vi "Begin.vi"(8 "error in":errorcluster) -> (0 "error out":errorcluster)   [LabVIEW 2017]
doc: "Called before other user functions, this VI is expected to open initial I/O refnums, load in file data, and do all program initialization. Notice that the <B>error out</B> terminal is simply used for data flow. Wiring it to other structures or subVIs ensures that this VI runs first."
uses:
  <vilib>/Rock Robotics/WPI/DriverStation/WPI_DriverStationRobotMode2.ctl
  <vilib>/Rock Robotics/WPI/Joystick/WPI_JoystickDeviceEnum.ctl
  <vilib>/Rock Robotics/WPI/ThirdParty/Phoenix-LabVIEW/Motor Controller/Controls/CTRE_Phoenix_MotorControl_NeutralMode.ctl
  <vilib>/Rock Robotics/WPI/ThirdParty/Phoenix-LabVIEW/Motor Controller/Controls/CTRE_Phoenix_MotorControl_ControlMode.ctl
  <vilib>/Rock Robotics/SystemInterfaces/spilib/spi_bus.ctl
  <vilib>/Rock Robotics/WPI/ThirdParty/Phoenix-LabVIEW/Motor Controller/Controls/CTRE_Phoenix_MotorControl_FeedbackDevice.ctl
  <vilib>/Rock Robotics/WPI/Solenoid/WPI_SolenoidChannel.ctl
  <vilib>/Rock Robotics/WPI/Solenoid/WPI_SolenoidValue.ctl
  Robot Global Data.vi
  <vilib>/Rock Robotics/Network Tables/NT Write String Array.vi
  <vilib>/Rock Robotics/WPI/RobotDrive/WPI_RobotDriveOpen2MotorWithExistingMotors.vi
  <vilib>/Rock Robotics/WPI/Solenoid/WPI_SolenoidOpenDouble.vi
  <vilib>/Rock Robotics/WPI/Solenoid/WPI_SolenoidSetEnum.vi
  <vilib>/Rock Robotics/WPI/Utilities/WPI_GetSetVariantRefNum.vi
  <vilib>/Rock Robotics/Network Tables/NT Write String.vi
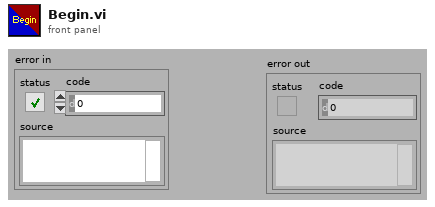
[diagram p1: front panel]
types:
  T1 = typedef "WPI_DriverStationRobotMode2.ctl" = enum16{"Autonomous Disabled", "Autonomous Enabled", "Teleop Disabled", "Teleop Enabled", "Disconnected", "Finish", "Test Disabled", "Test Enabled", "Emergency Stopped"}
  T2 = typedef "WPI_JoystickDeviceEnum.ctl" = enum16{"USB 0", "USB 1", "USB 2", "USB 3", "USB 4", "USB 5"}
  T3 = typedef "CTRE_Phoenix_MotorControl_NeutralMode.ctl" = enum8{"EEPROMSetting", "Override to Coast", "Override to Brake"}
  T4 = typedef "spi_bus.ctl" = enum16{"SPI On-Board, CS0", "SPI On-Board, CS1", "SPI On-Board, CS2", "SPI On-Board, CS3", "SPI MXP", "Invalid"}
  T5 = typedef "WPI_SolenoidValue.ctl" = enum16{"Off", "On", "Forward", "Reverse"}
  T6 = typedef "WPI_SolenoidChannel.ctl" = enum8{"Solenoid 0", "Solenoid 1", "Solenoid 2", "Solenoid 3", "Solenoid 4", "Solenoid 5", "Solenoid 6", "Solenoid 7", "Invalid"}
  T7 = typedef "WPI_JoystickDevRef.ctl" = cluster{"Device":T2}
  T8 = typedef "CTRE_Phoenix_MotorControl_ControlMode.ctl" = u16
  T9 = typedef "WPI_MotorControlDeviceRef.ctl" = cluster{"DeviceStatus":errorcluster, "Type":T10, "PWM":cluster{"PWM Channel":T11, "DeadBand":T12}, "CAN":cluster{"Device Number":u8, "SetOutput VI Ref":variant, "GetOutput VI Ref":variant, "Enable VI Ref":variant, "Disable VI Ref":variant, "Data":variant}, "Invert":bool, "DIO PWM":cluster{"PWM \"Enable\" Channel":T11, "DIOChannel":T13, "PWM Rate":dbl}}
  T10 = typedef "WPI_MotorControlType.ctl" = enum16{"PWM", "CAN", "DIO PWM"}
  T11 = typedef "FPGA_DIOPWMChannel.ctl" = enum8{"PWM 0", "PWM 1", "PWM 2", "PWM 3", "PWM 4", "PWM 5", "PWM 6", "PWM 7", "PWM 8", "PWM 9", "PWM MXP 0", "PWM MXP 1", "PWM MXP 2", "PWM MXP 3", "PWM MXP 4", "PWM MXP 5", "PWM MXP 6", "PWM MXP 7", "PWM MXP 8", "PWM MXP 9", "Invalid"}
  T12 = typedef "WPI_PWMDeadband.ctl" = cluster{"Name":string, "maxPositivePwm":i32, "minPositivePwm":i32, "centerPwm":i32, "maxNegativePwm":i32, "minNegativePwm":i32, "angularRange":u16}
  T13 = typedef "FPGA_DIOChannel.ctl" = enum8{"DIO 0", "DIO 1", "DIO 2", "DIO 3", "DIO 4", "DIO 5", "DIO 6", "DIO 7", "DIO 8", "DIO 9", "DIO MXP 0", "DIO MXP 1", "DIO MXP 2", "DIO MXP 3", "DIO MXP 4", "DIO MXP 5", "DIO MXP 6", "DIO MXP 7", "DIO MXP 8", "DIO MXP 9", "DIO MXP 10", "DIO MXP 11", "DIO MXP 12", "DIO MXP 13", "DIO MXP 14", "DIO MXP 15", "SPI Port CS1", "SPI Port CS2", "SPI Port CS3", "SPI Port MISO", "SPI Port MOSI", "Invalid"}
  T14 = typedef "WPI_RobotDriveDevRef.ctl" = cluster{"DevStatus":errorcluster, "Motors[]":T9[], "Square Inputs":bool, "Max Output":dbl}
  T15 = typedef "WPI_GyroDevRef.ctl" = cluster{"DevStatus":errorcluster, "Analog Channel":T16, "Gain (VoltsPerDegree/Second)":dbl, "Gyro Type":enum16{"Analog", "XRS450"}, "Handle":i32, "SPI Bus":T4, "Device Found":bool, "Sample Rate":dbl, "Calibrate On Open":bool, "Offset":dbl}
  T16 = typedef "FPGA_AIChannel.ctl" = enum8{"AI 0", "AI 1", "AI 2", "AI 3", "AI MXP 0", "AI MXP 1", "AI MXP 2", "AI MXP 3", "Invalid"}
  T17 = typedef "CTRE_Phoenix_MotorControl_FeedbackDevice.ctl" = i8
  T18 = typedef "WPI_SolenoidDevRef.ctl" = cluster{"DevStatus":errorcluster, "Pneumatics Control Module":u8, "Forward Solenoid Channel":T6, "Reverse Solenoid Channel":T6}
  T19 = typedef "WPI_CompressorDevRef.ctl" = cluster{"DevStatus":errorcluster, "Pneumatics Control Module":u8}
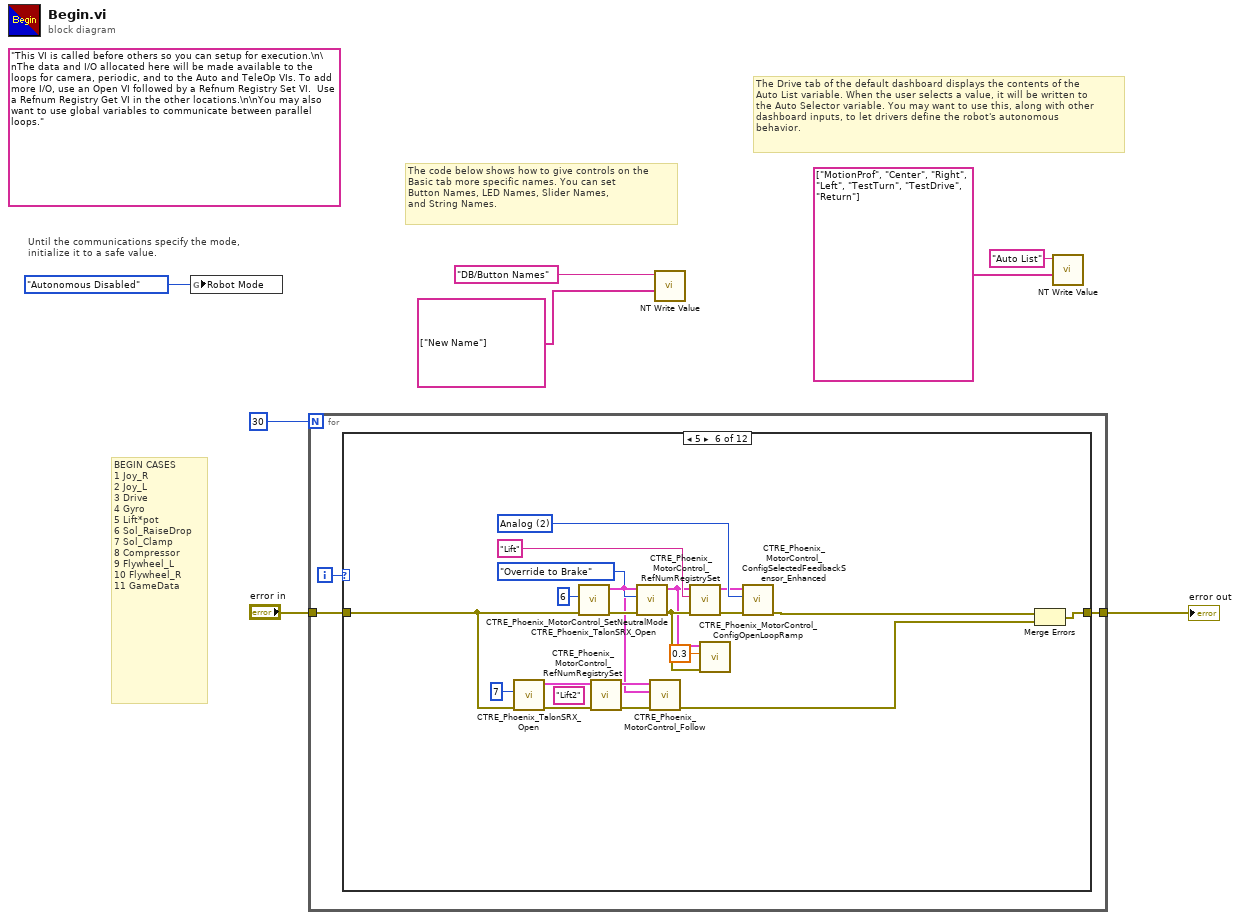
[diagram p0: block diagram]
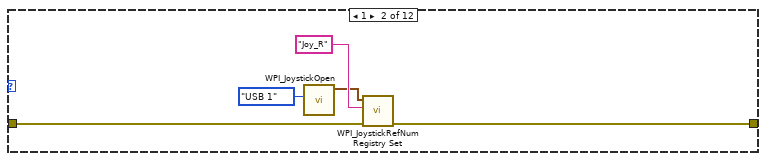
[diagram p3: hidden frame]
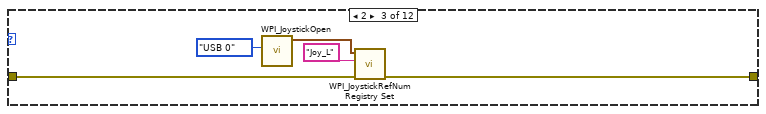
[diagram p4: hidden frame]
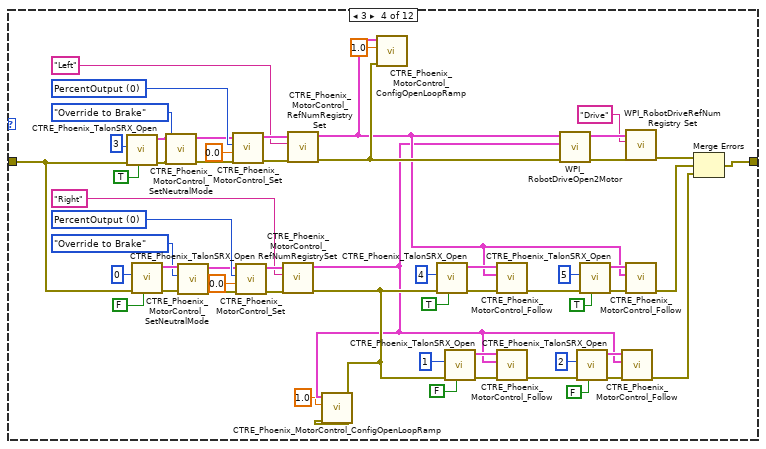
[diagram p5: hidden frame]
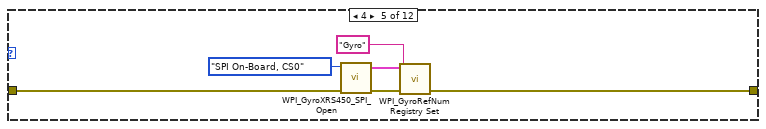
[diagram p6: hidden frame]
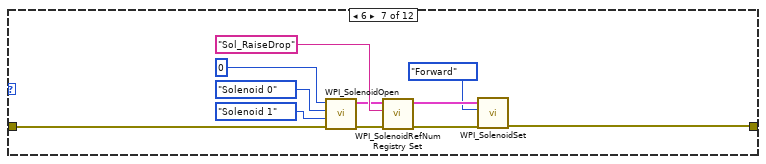
[diagram p7: hidden frame]
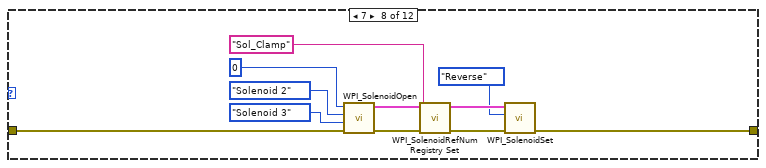
[diagram p8: hidden frame]
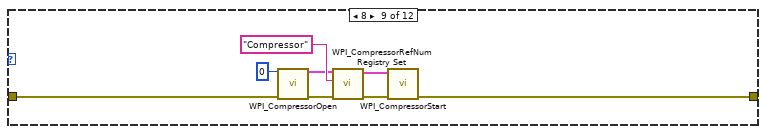
[diagram p9: hidden frame]
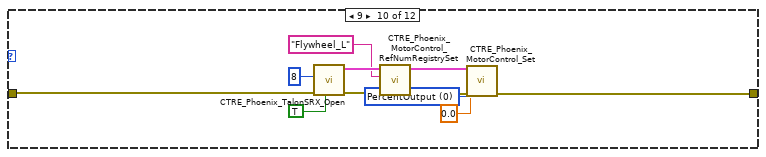
[diagram p10: hidden frame]
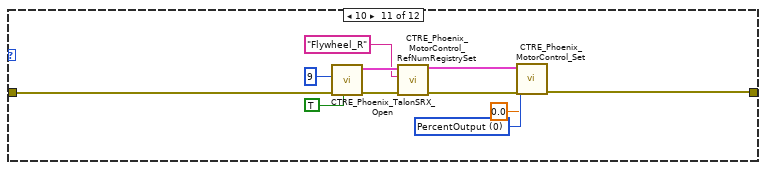
[diagram p11: hidden frame]
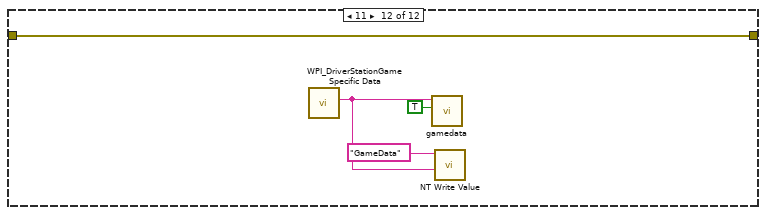
[diagram p12: hidden frame]
diagram:
  (unwired) "This VI is called before others so you can setup for execution.\n\nThe data and I/O allocated here will be made available to the loops for camera, periodic, and to the Auto and TeleOp VIs. To add more I/O, use an Open VI followed by a Refnum Registry Set VI.  Use a Refnum Registry Get VI in the other locations.\n\nYou may also want to use global variables to communicate between parallel loops."
  # "BEGIN CASES\n1 Joy_R\n2 Joy_L\n3 Drive\n4 Gyro\n5 Lift*pot\n6 Sol_RaiseDrop\n7 Sol_Clamp\n8 Compressor\n9 Flywheel_L\n10 Flywheel_R\n11 GameData"
  # "The Drive tab of the default dashboard displays the contents of the\nAuto List variable. When the user selects a value, it will be written to\nthe Auto Selector variable. You may want to use this, along with other\ndashboard inputs, to let drivers define the robot's autonomous\nbehavior."
  # "The code below shows how to give controls on the\nBasic tab more specific names. You can set\nButton Names, LED Names, Slider Names,\nand String Names."
  # "Until the communications specify the mode,\ninitialize it to a safe value."
  n1 = global write "Robot Global Data.vi" "Robot Mode"(WPI_DriverStationRobotMode2."Autonomous Disabled" ("Robot Mode")) -> ()
  n2 = for {
    N: 30 -> [_]
    tunnel: "error in" -> [w10]
    tunnel: [w9] -> w1
    i -> [w11]
    n3 = case shown="5" w11 {
      tunnel: w10 -> [w12 w16 w21 w39 w84 w86 w116 w122 w135 w146 w157 w161]
      tunnel: [w12 w15 w20 w78 w83 w87 w106 w118 w128 w139 w149 w161] -> w9
      frame 0, Default {
      }
      frame 1 {
        n4 = call <vilib>:"WPI_JoystickOpen.vi"("JoystickDevice"=WPI_JoystickDeviceEnum."USB 1") -> ("JoystickDevRef"=w14:T7)  [unwired: 10 in]
        n5 = call <vilib>:"WPI_JoystickRefNum Registry Set.vi"("error in (no error)"=w16, "refnum name"="Joy_R", "JoystickDevRef"=w14) -> ("error out"=w15:errorcluster)  [unwired: 7 in, 1 out]
      }
      frame 2 {
        n6 = call <vilib>:"WPI_JoystickOpen.vi"("JoystickDevice"=WPI_JoystickDeviceEnum."USB 0") -> ("JoystickDevRef"=w19:T7)  [unwired: 10 in]
        n7 = call <vilib>:"WPI_JoystickRefNum Registry Set.vi"("error in (no error)"=w21, "refnum name"="Joy_L", "JoystickDevRef"=w19) -> ("error out"=w20:errorcluster)  [unwired: 7 in, 1 out]
      }
      frame 3 {
        w61 = T8 0 items=["PercentOutput"=0, "Position"=1, "Velocity"=2, "Current"=3, "Follower"=5, "MotionProfile"=6, "MotionMagic"=7, "MotionMagicArc"=8, "MotionProfileArc"=10, "Disabled"=15] ("Control Mode")
        w71 = T8 0 items=["PercentOutput"=0, "Position"=1, "Velocity"=2, "Current"=3, "Follower"=5, "MotionProfile"=6, "MotionMagic"=7, "MotionMagicArc"=8, "MotionProfileArc"=10, "Disabled"=15] ("Control Mode")
        n8 = call <vilib>:"CTRE_Phoenix_TalonSRX_Open.vi"("Invert"=TRUE, "error in"=w39, "Device Number"=u8 3) -> ("error out"=w77:errorcluster, "CAN Talon SRX Ref"=w76:T9)  [unwired: 7 in]
        n9 = call <vilib>:"CTRE_Phoenix_TalonSRX_Open.vi"("Invert"=FALSE, "error in"=w39, "Device Number"=u8 0) -> ("error out"=w67:errorcluster, "CAN Talon SRX Ref"=w66:T9)  [unwired: 7 in]
        n10 = call <vilib>:"CTRE_Phoenix_MotorControl_SetNeutralMode.vi"("error in (no error)"=w77, "Motor Control Neutral Mode"=CTRE_Phoenix_MotorControl_NeutralMode."Override to Brake", "PhoenixMotorControlDevRef"=w76) -> ("error out"=w26:errorcluster, "PhoenixMotorControlDevRef"=w27:T9)  [unwired: 7 in]
        n11 = call <vilib>:"CTRE_Phoenix_MotorControl_SetNeutralMode.vi"("error in (no error)"=w67, "Motor Control Neutral Mode"=CTRE_Phoenix_MotorControl_NeutralMode."Override to Brake", "PhoenixMotorControlDevRef"=w66) -> ("error out"=w25:errorcluster, "PhoenixMotorControlDevRef"=w28:T9)  [unwired: 7 in]
        n12 = call <vilib>:"CTRE_Phoenix_MotorControl_Set.vi"("error in (no error)"=w26, "Output"=0.0, "Control Mode"=w71, "PhoenixMotorControlDevRef"=w27) -> ("error out"=w74:errorcluster, "PhoenixMotorControlDevRef"=w75:T9)  [unwired: 6 in]
        n13 = call <vilib>:"CTRE_Phoenix_MotorControl_Set.vi"("error in (no error)"=w25, "Output"=0.0, "Control Mode"=w61, "PhoenixMotorControlDevRef"=w28) -> ("error out"=w64:errorcluster, "PhoenixMotorControlDevRef"=w65:T9)  [unwired: 6 in]
        n14 = call <vilib>:"CTRE_Phoenix_MotorControl_RefNumRegistrySet.vi"("error in (no error)"=w64, "refnum name"="Right", "PhoenixMotorControlDevRef"=w65) -> ("error out"=w30:errorcluster, "PhoenixMotorControlDevRef"=w29:T9)  [unwired: 7 in]
        n15 = call <vilib>:"CTRE_Phoenix_MotorControl_RefNumRegistrySet.vi"("error in (no error)"=w74, "refnum name"="Left", "PhoenixMotorControlDevRef"=w75) -> ("error out"=w32:errorcluster, "PhoenixMotorControlDevRef"=w31:T9)  [unwired: 7 in]
        n16 = call <vilib>:"CTRE_Phoenix_MotorControl_ConfigOpenLoopRamp.vi"("error in (no error)"=w30, "secondsFromNeutralToFull"=1.0, "PhoenixMotorControlDevRef"=w29) -> ()  [unwired: 7 in, 2 out]
        n17 = call <vilib>:"CTRE_Phoenix_MotorControl_ConfigOpenLoopRamp.vi"("error in (no error)"=w32, "secondsFromNeutralToFull"=1.0, "PhoenixMotorControlDevRef"=w31) -> ()  [unwired: 7 in, 2 out]
        n18 = call <vilib>:"CTRE_Phoenix_TalonSRX_Open.vi"("Invert"=TRUE, "error in"=w30, "Device Number"=u8 4) -> ("error out"=w37:errorcluster, "CAN Talon SRX Ref"=w54:T9)  [unwired: 7 in]
        n19 = call <vilib>:"CTRE_Phoenix_TalonSRX_Open.vi"("Invert"=FALSE, "error in"=w30, "Device Number"=u8 1) -> ("error out"=w51:errorcluster, "CAN Talon SRX Ref"=w50:T9)  [unwired: 7 in]
        n20 = call <vilib>:"CTRE_Phoenix_MotorControl_Follow.vi"("error in (no error)"=w37, "Master Controller to Follow"=w31, "PhoenixMotorControlDevRef"=w54) -> ("error out"=w36:errorcluster)  [unwired: 7 in, 1 out]
        n21 = call <vilib>:"CTRE_Phoenix_MotorControl_Follow.vi"("error in (no error)"=w51, "Master Controller to Follow"=w29, "PhoenixMotorControlDevRef"=w50) -> ("error out"=w35:errorcluster)  [unwired: 7 in, 1 out]
        n22 = call-poly <vilib>:"WPI_RobotDriveOpen2Motor.vi"("error in (no error)"=w32, "Right Motor Dev Ref"=w29, "Left Motor Dev Ref"=w31) -> ("error out"=w56:errorcluster, "RobotDriveDevRef"=w57:T14)  [unwired: 7 in]
        n23 = call <vilib>:"CTRE_Phoenix_TalonSRX_Open.vi"("Invert"=FALSE, "error in"=w35, "Device Number"=u8 2) -> ("error out"=w43:errorcluster, "CAN Talon SRX Ref"=w42:T9)  [unwired: 7 in]
        n24 = call <vilib>:"CTRE_Phoenix_TalonSRX_Open.vi"("Invert"=TRUE, "error in"=w36, "Device Number"=u8 5) -> ("error out"=w47:errorcluster, "CAN Talon SRX Ref"=w46:T9)  [unwired: 7 in]
        n25 = call <vilib>:"CTRE_Phoenix_MotorControl_Follow.vi"("error in (no error)"=w43, "Master Controller to Follow"=w29, "PhoenixMotorControlDevRef"=w42) -> ("error out"=w33:errorcluster)  [unwired: 7 in, 1 out]
        n26 = call <vilib>:"WPI_RobotDriveRefNum Registry Set.vi"("error in (no error)"=w56, "refnum name"="Drive", "RobotDriveDevRef"=w57) -> ("error out"=w38:errorcluster)  [unwired: 7 in, 1 out]
        n27 = call <vilib>:"CTRE_Phoenix_MotorControl_Follow.vi"("error in (no error)"=w47, "Master Controller to Follow"=w31, "PhoenixMotorControlDevRef"=w46) -> ("error out"=w34:errorcluster)  [unwired: 7 in, 1 out]
        n28 = Merge Errors(w38, w34, w33) -> (w78:errorcluster)
      }
      frame 4 {
        n29 = call <vilib>:"WPI_GyroXRS450_SPI_Open.vi"("error in"=w84, "SPI Bus"=spi_bus."SPI On-Board, CS0") -> ("error out"=w82:errorcluster, "GyroDevRef"=w81:T15)  [unwired: 7 in, 1 out]
        n30 = call <vilib>:"WPI_GyroRefNum Registry Set.vi"("error in (no error)"=w82, "refnum name"="Gyro", "GyroDevRef"=w81) -> ("error out"=w83:errorcluster)  [unwired: 7 in, 1 out]
      }
      frame 5 {
        w103 = T17 2 items=["None"=-1, "QuadEncoder"=0, "Analog"=2, "Tachometer"=4, "Pulse Width Encoded Position"=8, "Sensor Sum (S0 + S1)"=9, "Sensor Difference (D0 - D1)"=10, "Remote Source 0"=11, "Remote Source 1"=12, "Software Emulated"=15] ("Feedback Device")
        n31 = call <vilib>:"CTRE_Phoenix_TalonSRX_Open.vi"("error in"=w86, "Device Number"=7) -> ("error out"=w93:errorcluster, "CAN Talon SRX Ref"=w95:T9)  [unwired: 8 in]
        n32 = call <vilib>:"CTRE_Phoenix_TalonSRX_Open.vi"("error in"=w86, "Device Number"=u8 6) -> ("error out"=w100:errorcluster, "CAN Talon SRX Ref"=w91:T9)  [unwired: 8 in]
        n33 = call <vilib>:"CTRE_Phoenix_MotorControl_RefNumRegistrySet.vi"("error in (no error)"=w93, "refnum name"="Lift2", "PhoenixMotorControlDevRef"=w95) -> ("error out"=w90:errorcluster, "PhoenixMotorControlDevRef"=w92:T9)  [unwired: 7 in]
        n34 = call <vilib>:"CTRE_Phoenix_MotorControl_SetNeutralMode.vi"("error in (no error)"=w100, "Motor Control Neutral Mode"=CTRE_Phoenix_MotorControl_NeutralMode."Override to Brake", "PhoenixMotorControlDevRef"=w91) -> ("error out"=w98:errorcluster, "PhoenixMotorControlDevRef"=w97:T9)  [unwired: 7 in]
        n35 = call <vilib>:"CTRE_Phoenix_MotorControl_Follow.vi"("error in (no error)"=w90, "Master Controller to Follow"=w91, "PhoenixMotorControlDevRef"=w92) -> ("error out"=w88:errorcluster)  [unwired: 7 in, 1 out]
        n36 = call <vilib>:"CTRE_Phoenix_MotorControl_RefNumRegistrySet.vi"("error in (no error)"=w98, "refnum name"="Lift", "PhoenixMotorControlDevRef"=w97) -> ("error out"=w102:errorcluster, "PhoenixMotorControlDevRef"=w101:T9)  [unwired: 7 in]
        n37 = call <vilib>:"CTRE_Phoenix_MotorControl_ConfigOpenLoopRamp.vi"("error in (no error)"=w98, "secondsFromNeutralToFull"=0.3, "PhoenixMotorControlDevRef"=w97) -> ()  [unwired: 7 in, 2 out]
        n38 = call <vilib>:"CTRE_Phoenix_MotorControl_ConfigSelectedFeedbackSensor_Enhanced.vi"("error in (no error)"=w102, "Feedback Device"=w103, "PhoenixMotorControlDevRef"=w101) -> ("error out"=w89:errorcluster)  [unwired: 7 in, 1 out]
        n39 = Merge Errors(w89, w88) -> (w87:errorcluster)
      }
      frame 6 {
        n40 = call-poly <vilib>:"WPI_SolenoidOpen.vi"("error in (no error)"=w116, "Reverse Solenoid Channel"=WPI_SolenoidChannel."Solenoid 1", "Forward Solenoid Channel"=WPI_SolenoidChannel."Solenoid 0" ("Solenoid Channel"), "Pneumatics Control Module (0)"=u8 0) -> ("error out"=w112:errorcluster, "SolenoidDevRef"=w114:T18)  [unwired: 6 in]
        n41 = call <vilib>:"WPI_SolenoidRefNum Registry Set.vi"("error in (no error)"=w112, "refnum name"="Sol_RaiseDrop", "SolenoidDevRef"=w114) -> ("error out"=w109:errorcluster, "SolenoidDevRef"=w108:T18)  [unwired: 7 in]
        n42 = call-poly <vilib>:"WPI_SolenoidSet.vi"("error in (no error)"=w109, "Value"=WPI_SolenoidValue."Forward", "SolenoidDevRef"=w108) -> ("error out"=w106:errorcluster)  [unwired: 7 in, 1 out]
      }
      frame 7 {
        n43 = call-poly <vilib>:"WPI_SolenoidOpen.vi"("error in (no error)"=w122, "Reverse Solenoid Channel"=WPI_SolenoidChannel."Solenoid 3", "Forward Solenoid Channel"=WPI_SolenoidChannel."Solenoid 2" ("Solenoid Channel"), "Pneumatics Control Module (0)"=u8 0) -> ("error out"=w127:errorcluster, "SolenoidDevRef"=w126:T18)  [unwired: 6 in]
        n44 = call <vilib>:"WPI_SolenoidRefNum Registry Set.vi"("error in (no error)"=w127, "refnum name"="Sol_Clamp", "SolenoidDevRef"=w126) -> ("error out"=w119:errorcluster, "SolenoidDevRef"=w120:T18)  [unwired: 7 in]
        n45 = call-poly <vilib>:"WPI_SolenoidSet.vi"("error in (no error)"=w119, "Value"=WPI_SolenoidValue."Reverse", "SolenoidDevRef"=w120) -> ("error out"=w118:errorcluster)  [unwired: 7 in, 1 out]
      }
      frame 8 {
        n46 = call <vilib>:"WPI_CompressorOpen.vi"("Pneumatics Control Module (0)"=u8 0, "error in (no error)"=w135) -> ("CompressorDevRef"=w132:T19, "error out"=w130:errorcluster)  [unwired: 12 in]
        n47 = call <vilib>:"WPI_CompressorRefNum Registry Set.vi"("error in (no error)"=w130, "refnum name"="Compressor", "CompressorDevRef"=w132) -> ("error out"=w131:errorcluster, "CompressorDevRef"=w133:T19)  [unwired: 7 in]
        n48 = call <vilib>:"WPI_CompressorStart.vi"("error in (no error)"=w131, "CompressorDevRef"=w133) -> ("error out"=w128:errorcluster)  [unwired: 8 in, 1 out]
      }
      frame 9 {
        w138 = T8 0 items=["PercentOutput"=0, "Position"=1, "Velocity"=2, "Current"=3, "Follower"=5, "MotionProfile"=6, "MotionMagic"=7, "MotionMagicArc"=8, "MotionProfileArc"=10, "Disabled"=15] ("Control Mode")
        n49 = call <vilib>:"CTRE_Phoenix_TalonSRX_Open.vi"("Invert"=TRUE, "error in"=w146, "Device Number"=u8 8) -> ("error out"=w144:errorcluster, "CAN Talon SRX Ref"=w145:T9)  [unwired: 7 in]
        n50 = call <vilib>:"CTRE_Phoenix_MotorControl_RefNumRegistrySet.vi"("error in (no error)"=w144, "refnum name"="Flywheel_L", "PhoenixMotorControlDevRef"=w145) -> ("error out"=w140:errorcluster, "PhoenixMotorControlDevRef"=w136:T9)  [unwired: 7 in]
        n51 = call <vilib>:"CTRE_Phoenix_MotorControl_Set.vi"("error in (no error)"=w140, "Output"=0.0, "Control Mode"=w138, "PhoenixMotorControlDevRef"=w136) -> ("error out"=w139:errorcluster)  [unwired: 6 in, 1 out]
      }
      frame 10 {
        w151 = T8 0 items=["PercentOutput"=0, "Position"=1, "Velocity"=2, "Current"=3, "Follower"=5, "MotionProfile"=6, "MotionMagic"=7, "MotionMagicArc"=8, "MotionProfileArc"=10, "Disabled"=15] ("Control Mode")
        n52 = call <vilib>:"CTRE_Phoenix_TalonSRX_Open.vi"("Invert"=TRUE, "error in"=w157, "Device Number"=u8 9) -> ("error out"=w155:errorcluster, "CAN Talon SRX Ref"=w156:T9)  [unwired: 7 in]
        n53 = call <vilib>:"CTRE_Phoenix_MotorControl_RefNumRegistrySet.vi"("error in (no error)"=w155, "refnum name"="Flywheel_R", "PhoenixMotorControlDevRef"=w156) -> ("error out"=w148:errorcluster, "PhoenixMotorControlDevRef"=w147:T9)  [unwired: 7 in]
        n54 = call <vilib>:"CTRE_Phoenix_MotorControl_Set.vi"("error in (no error)"=w148, "Output"=0.0, "Control Mode"=w151, "PhoenixMotorControlDevRef"=w147) -> ("error out"=w149:errorcluster)  [unwired: 6 in, 1 out]
      }
      frame 11 {
        n55 = call <vilib>:"WPI_DriverStationGame Specific Data.vi"() -> ("Game Specific Data"=w159:string)  [unwired: 11 in]
        n56 = call "gamedata.vi"("set(T)/get(F) 2"=TRUE, "String 2"=w159) -> ()  [unwired: 9 in, 1 out]
        n57 = call-poly <vilib>:"NT Write Value.vi"("String"=w159, "Name"="GameData") -> ()  [unwired: 9 in, 1 out]
      }
    }
  }
  "error out" <- w1
  n58 = call-poly <vilib>:"NT Write Value.vi"("String Array"=string[] ["New Name"], "Name"="DB/Button Names") -> ()  [unwired: 9 in, 1 out]
  n59 = call-poly <vilib>:"NT Write Value.vi"("String Array"=string[] ["MotionProf", "Center", "Right", "Left", "TestTurn", "TestDrive", "Return"], "Name"="Auto List") -> ()  [unwired: 9 in, 1 out]
